vi "Configure Pulse Mode.vi"(0 "VISA resource name":refnum<visa-resource-name>, 1 "Pulse AC Frequency (50 Hz)":dbl=50.0 min=43.0 max=1200.0 format="%.3g", 2 "Pulse Voltage":T1 {"Pulse DC Voltage (0 V)" format="%.3g"; "Pulse AC Voltage (0 V)" format="%.3g"}, 5 "Pulse Sync (0: Immediate)":i32(ring) items=["Immediate", "Phase"], 7 "Pulse Phase (0.0 degrees)":dbl min=0.0 max=359.7 format="%.1g", 9 "Pulse Period (0 ms)":u32 max=100000, 11 "error in (no error)":errorcluster, 12 "Pulse Duty (0 %)":u32 max=100, 13 "Pulse Count (1)":u32=1 max=99) -> (4 "VISA resource name out":refnum<visa-resource-name>, 15 "error out":errorcluster)   [LabVIEW 2018, in "BK Precision 983X Series.lvlib"]
doc: "Configures all the parameters for pulse output mode.\n\nNote: Run <b>Configure Output Mode.vi</b> first to set the instrument to Pulse Mode before running this vi."
uses:
  <instrlib>/BK Precision 983X Series/BK Precision 983X Series.lvlib
panel:
  # "ms"
  # "%"
  # "V"
  # "V"
  # "degree"
  # "Hz"
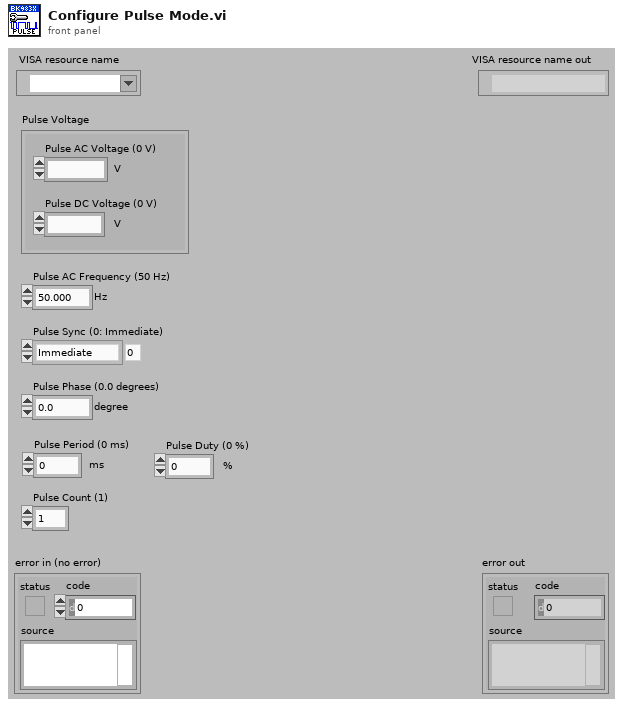
[diagram p1: front panel]
types:
  T1 = cluster{"Pulse AC Voltage (0 V)":dbl, "Pulse DC Voltage (0 V)":dbl}
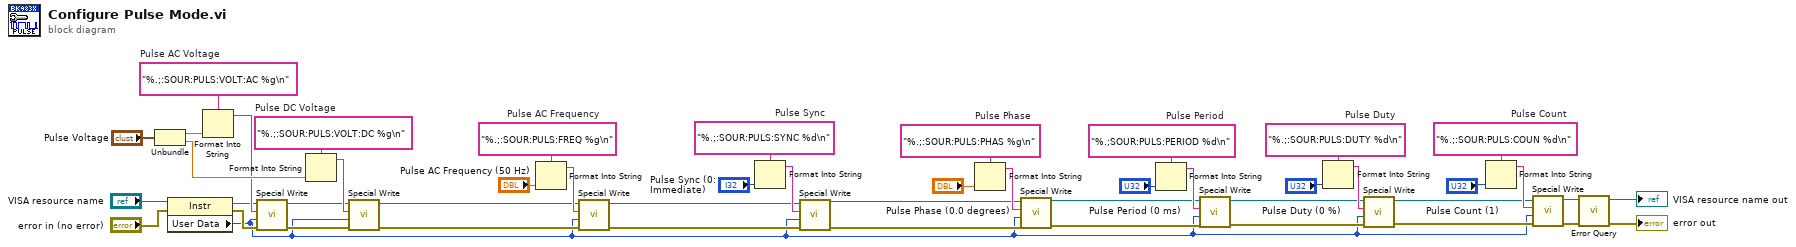
[diagram p0: block diagram]
diagram:
  w26 = "%.;SOUR:PULS:PERIOD %d\n"  # Pulse Period
  w40 = "%.;:SOUR:PULS:DUTY %d\n"  # Pulse Duty
  w41 = "%.;:SOUR:PULS:PHAS %g\n"  # Pulse Phase
  w42 = "%.;:SOUR:PULS:SYNC %d\n"  # Pulse Sync
  w43 = "%.;:SOUR:PULS:VOLT:DC %g\n"  # Pulse DC Voltage
  w44 = "%.;:SOUR:PULS:COUN %d\n"  # Pulse Count
  w45 = "%.;:SOUR:PULS:FREQ %g\n"  # Pulse AC Frequency
  w46 = "%.;:SOUR:PULS:VOLT:AC %g\n"  # Pulse AC Voltage
  n1 = Unbundle("Pulse Voltage") -> ("Pulse AC Voltage (0 V)"=w29:dbl, "Pulse DC Voltage (0 V)"=w28:dbl)
  n2 = property class="Instr"(reference="VISA resource name", error in="error in (no error)") -> (reference out=w23:refnum<visa-resource-name>, error out=w22:errorcluster, "User Data"=w1:u32)
  n3 = Format Into String(format string=w46, w29) -> (resulting string=w24:string)  [unwired: 2 in, 1 out]
  n4 = call <instrlib>:"Special Write.vi"("error in (no error)"=w22, "Delay (0 ms)"=w1, "Input String"=w24, "VISA resource name"=w23) -> ("error out"=w19:errorcluster, "VISA resource name out"=w20:refnum<visa-resource-name>)  [unwired: 6 in]
  n5 = Format Into String(format string=w43, w28) -> (resulting string=w21:string)  [unwired: 2 in, 1 out]
  n6 = call <instrlib>:"Special Write.vi"("error in (no error)"=w19, "Delay (0 ms)"=w1, "Input String"=w21, "VISA resource name"=w20) -> ("error out"=w16:errorcluster, "VISA resource name out"=w17:refnum<visa-resource-name>)  [unwired: 6 in]
  n7 = Format Into String(format string=w45, "Pulse AC Frequency (50 Hz)") -> (resulting string=w18:string)  [unwired: 2 in, 1 out]
  n8 = call <instrlib>:"Special Write.vi"("error in (no error)"=w16, "Delay (0 ms)"=w1, "Input String"=w18, "VISA resource name"=w17) -> ("error out"=w13:errorcluster, "VISA resource name out"=w14:refnum<visa-resource-name>)  [unwired: 6 in]
  n9 = Format Into String(format string=w42, "Pulse Sync (0: Immediate)") -> (resulting string=w15:string)  [unwired: 2 in, 1 out]
  n10 = call <instrlib>:"Special Write.vi"("error in (no error)"=w13, "Delay (0 ms)"=w1, "Input String"=w15, "VISA resource name"=w14) -> ("error out"=w10:errorcluster, "VISA resource name out"=w11:refnum<visa-resource-name>)  [unwired: 6 in]
  n11 = Format Into String(format string=w41, "Pulse Phase (0.0 degrees)") -> (resulting string=w12:string)  [unwired: 2 in, 1 out]
  n12 = call <instrlib>:"Special Write.vi"("error in (no error)"=w10, "Delay (0 ms)"=w1, "Input String"=w12, "VISA resource name"=w11) -> ("error out"=w7:errorcluster, "VISA resource name out"=w8:refnum<visa-resource-name>)  [unwired: 6 in]
  n13 = Format Into String(format string=w26, "Pulse Period (0 ms)") -> (resulting string=w9:string)  [unwired: 2 in, 1 out]
  n14 = call <instrlib>:"Special Write.vi"("error in (no error)"=w7, "Delay (0 ms)"=w1, "Input String"=w9, "VISA resource name"=w8) -> ("error out"=w4:errorcluster, "VISA resource name out"=w5:refnum<visa-resource-name>)  [unwired: 6 in]
  n15 = Format Into String(format string=w40, "Pulse Duty (0 %)") -> (resulting string=w6:string)  [unwired: 2 in, 1 out]
  n16 = call <instrlib>:"Special Write.vi"("error in (no error)"=w4, "Delay (0 ms)"=w1, "Input String"=w6, "VISA resource name"=w5) -> ("error out"=w2:errorcluster, "VISA resource name out"=w3:refnum<visa-resource-name>)  [unwired: 6 in]
  n17 = Format Into String(format string=w44, "Pulse Count (1)") -> (resulting string=w37:string)  [unwired: 2 in, 1 out]
  n18 = call <instrlib>:"Special Write.vi"("error in (no error)"=w2, "Delay (0 ms)"=w1, "Input String"=w37, "VISA resource name"=w3) -> ("error out"=w38:errorcluster, "VISA resource name out"=w39:refnum<visa-resource-name>)  [unwired: 6 in]
  n19 = call <instrlib>:"Error Query.vi"("error in (no error)"=w38, "VISA resource name"=w39) -> ("error out"=→"error out":errorcluster, "VISA resource name out"=→"VISA resource name out":refnum<visa-resource-name>)  [unwired: 6 in, 2 out]
